vi "ReadDefaultLibrarySize.vi"(8 "ErrorIn":errorcluster caption="Error In(no Error)", 11 "ReferenceIn":refnum<class "ErrorDefinitionSQLite.lvclass"> caption="Reference In") -> (0 "ErrorOut":errorcluster caption="Error Out", 2 "DefaultLibrarySize":i32, 3 "ReferenceOut":refnum<class "ErrorDefinitionSQLite.lvclass"> caption="Reference Out")   [LabVIEW 2018, in "ErrorDefinitionSQLite.lvclass"]
uses:
  ErrorDefinitionSQLite.lvclass
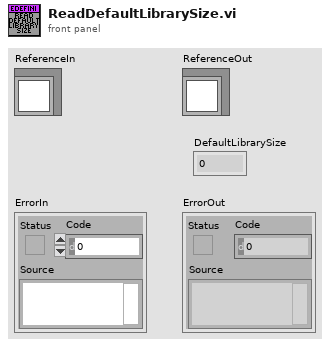
[diagram p1: front panel]
types:
  T1 = typedef "ErrorDefinitionSQLite.lvclass/ObjectAttributes.ctl" = cluster{"Path":path, "SQLiteRef":refnum<class "Connection.lvclass">, "EndOfRange":i32, "DefaultLibrarySize":i32, "StartOfRange":i32}
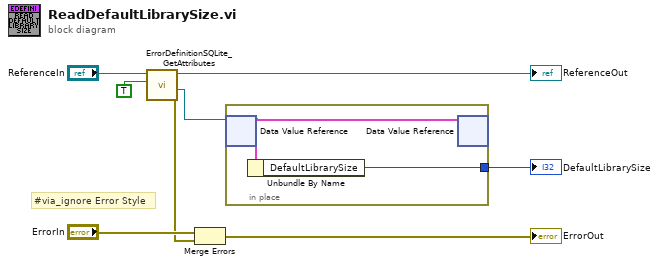
[diagram p0: block diagram]
diagram:
  # "#via_ignore Error Style"
  n1 = call "ErrorDefinitionSQLite_GetAttributes.vi"("OnlyGetDVRReference"=TRUE ("OnlyGetDvrReference(False)"), "Reference in"="ReferenceIn") -> ("ErrorOut"=w5:errorcluster, "DataRef"=w2:refnum<data-value>, "Reference out"=→"ReferenceOut":refnum<class "ErrorDefinitionSQLite.lvclass">)  [unwired: 6 in, 1 out]
  n2 = Merge Errors("ErrorIn", w5) -> (→"ErrorOut":errorcluster)
  n3 = in-place {
    in-place-border: [w10] -> w1
    n4 = in-place-dvr #1(w2) -> (w9:T1)  [unwired: 1 out]
    n5 = Unbundle By Name(w9) -> ("DefaultLibrarySize"=w10:i32)
    n6 = in-place-dvr #1(w9) -> ()  [unwired: 2 out]
  }
  "DefaultLibrarySize" <- w1
